vi "Add Subpalettes.vi"() -> ()   [LabVIEW 2019]
doc: "This VI shows how to add different types of subpalettes to an existing palette. Those types include:\n\n1. A standard .mnu file.\n2. A .mnu file within a .lvlib.\n3. A .lvlib with a default palette configured."
uses:
  <vilib>/Palette API/Palette Menu/Public Type Define/Palette type.ctl
  <vilib>/Palette API/Palette Menu/Public Type Define/Item.ctl
  <vilib>/Palette API/Palette Menu/Palette Menu.lvlib
panel:
  in  "short name (default lvlib)":string="default lvlib palette"
  in  "short name (lvlib)":string="lvlib palette"
  in  "short name (standard)":string="standard palette"
  # "Overview: Demonstrates the use of the Palette Editing VIs to add subpalettes to an existing palette.\nInstructions:\n1. Make sure you have already run the Create New Palette.vi example.\n2. Run this VI. It will add three new subpalettes to Functions > User Libraries > Palette API. See the block diagram for more information."
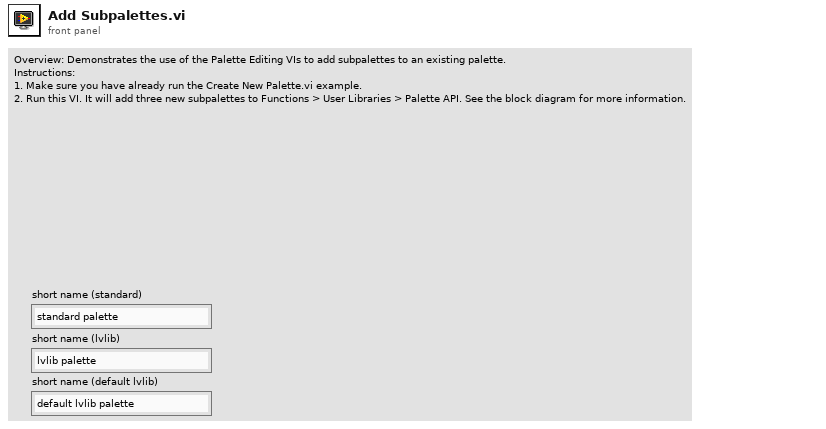
[diagram p1: front panel]
types:
  T1 = typedef "Palette Menu.lvlib/Item.ctl" = cluster{"item path":path, "library path":path, "use default lvlib palette":bool, "short name":string, "place VI contents":bool, "hide synchronized item":bool, "reserve spot for synch item":bool, "configure when placing VI contents":bool}
  T2 = typedef "Palette Menu.lvlib/Palette type.ctl" = i32
  T3 = typedef "Palette Menu.lvlib/Palette Data.ctl" = cluster{"display name":string, "view format":T4, "palette width":i16, "items":T5, "256 color icon":picture, "B&W color icon":picture, "help information":T6, "palette description":string, "synchronize information":T7}
  T4 = typedef "Palette Menu.lvlib/View Format.ctl" = u16
  T5 = typedef "Palette Menu.lvlib/Items.ctl" = T1[]
  T6 = typedef "Palette Menu.lvlib/Help Info.ctl" = cluster{"help tag":string, "help file path ":path}
  T7 = typedef "Palette Menu.lvlib/Synchronize Info.ctl" = cluster{"synchronize with directory":bool, "synchronize directory path":path}
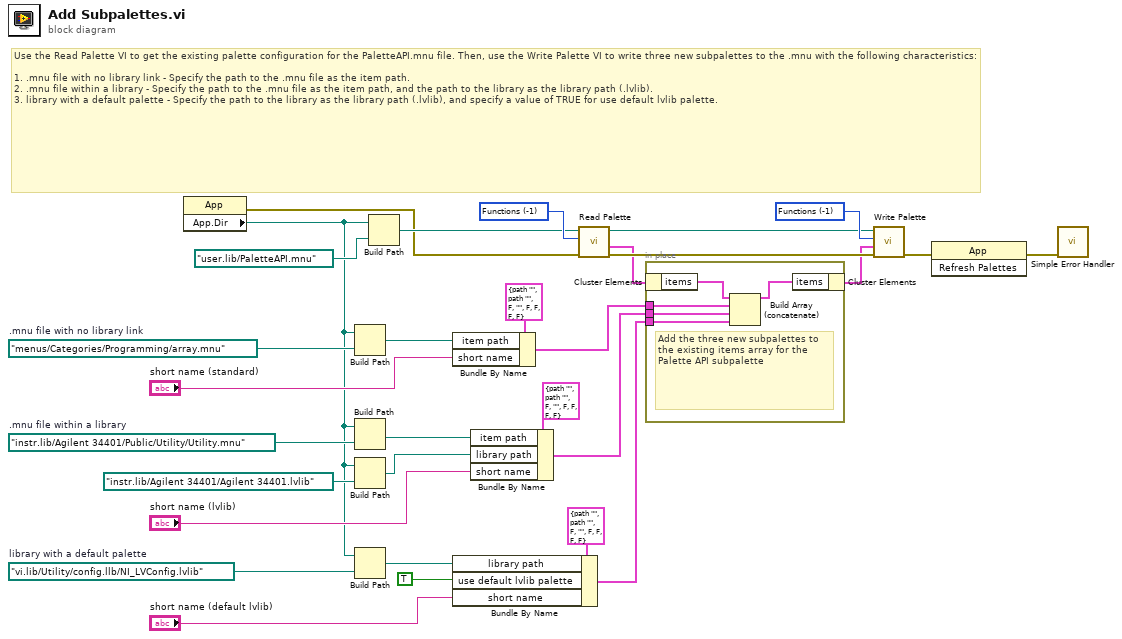
[diagram p0: block diagram]
diagram:
  w9 = path "vi.lib/Utility/config.llb/NI_LVConfig.lvlib"  # library with a default palette
  w12 = path "instr.lib/Agilent 34401/Public/Utility/Utility.mnu"  # .mnu file within a library
  w20 = path "menus/Categories/Programming/array.mnu"  # .mnu file with no library link
  w25 = T2 -1 items=["Functions"=-1, "Controls"=-2] ("palette type")
  w28 = T2 -1 items=["Functions"=-1, "Controls"=-2] ("palette type")
  # "Use the Read Palette VI to get the existing palette configuration for the PaletteAPI.mnu file. Then, use the Write Palette VI to write three new subpalettes to the .mnu with the following characteristics:\n\n1. .mnu file with no library link - Specify the path to the .mnu file as the item path.\n2. .mnu file within a library - Specify the path to the .mnu file as the item path, and the path to the library as the library path (.lvlib).\n3. library with a default palette - Specify the path to the library as the library path (.lvlib), and specify a value of TRUE for use default lvlib palette."
  n1 = property class="App"() -> (error out=w1:errorcluster, "App.Dir"=w2:path)  [unwired: 2 in, 1 out]
  n2 = Build Path(base path=w2, name or relative path=w20) -> (appended path=w19:path)
  n3 = Build Path(base path=w2, name or relative path=w12) -> (appended path=w13:path)
  n4 = Build Path(base path=w2, name or relative path=path "instr.lib/Agilent 34401/Agilent 34401.lvlib" ("String")) -> (appended path=w15:path)
  n5 = Build Path(base path=w2, name or relative path=w9) -> (appended path=w8:path)
  n6 = Build Path(base path=w2, name or relative path=path "user.lib/PaletteAPI.mnu") -> (appended path=w23:path)
  n7 = Bundle By Name(cluster=T1 {"item path"=path "", "library path"=path "", "use default lvlib palette"=FALSE, "short name"="", "place VI contents"=FALSE, "hide synchronized item"=FALSE, "reserve spot for synch item"=FALSE, "configure when placing VI contents"=FALSE} ("Items"), "item path"=w19, "short name"="short name (standard)") -> (w18:T1)
  n8 = Bundle By Name(cluster=T1 {"item path"=path "", "library path"=path "", "use default lvlib palette"=FALSE, "short name"="", "place VI contents"=FALSE, "hide synchronized item"=FALSE, "reserve spot for synch item"=FALSE, "configure when placing VI contents"=FALSE} ("Items"), "library path"=w8, "use default lvlib palette"=TRUE, "short name"="short name (default lvlib)") -> (w5:T1)
  n9 = Bundle By Name(cluster=T1 {"item path"=path "", "library path"=path "", "use default lvlib palette"=FALSE, "short name"="", "place VI contents"=FALSE, "hide synchronized item"=FALSE, "reserve spot for synch item"=FALSE, "configure when placing VI contents"=FALSE} ("Items"), "item path"=w13, "library path"=w15, "short name"="short name (lvlib)") -> (w6:T1)
  n10 = call <vilib>:"Read Palette.vi"("error in (no error)"=w1, "palette type"=w25, "palette path"=w23) -> ("error out"=w27:errorcluster, "palette data"=w4:T3, "duplicate palette path"=w26:path)  [unwired: 1 in, 5 out]
  n11 = in-place {
    in-place-border: w18 -> [w35]
    in-place-border: w6 -> [w34]
    in-place-border: w5 -> [w33]
    # "Add the three new subpalettes to the existing items array for the Palette API subpalette"
    n12 = in-place-cluster #1(w4) -> ("items"=w32:T5)
    n13 = Build Array (concatenate)(w32, w35, w34, w33) -> (w31:T5)
    n14 = in-place-cluster #1("items"=w31) -> (w3:T3)
  }
  n15 = call <vilib>:"Write Palette.vi"("error in (no error)"=w27, "palette data"=w3, "palette type"=w28, "palette path"=w26) -> ("error out"=w30:errorcluster)  [unwired: 1 in, 6 out]
  n16 = invoke class="App" method="Refresh Palettes"(error in=w30) -> (error out=w29:errorcluster)  [unwired: 2 in, 2 out]
  n17 = call <vilib>:"Simple Error Handler.vi"("error in (no error)"=w29) -> ()  [unwired: 1 in, 8 out]
